vi "Save param in PGserver.vi"(4 "Param row name 2":string, 6 "Param row name1":string, 7 "conninfo":T1={"host"="localhost", "port"="5432", "client_encoding"="WIN1251", "dbname"="system", "user"="postgres", "password"=""}, 8 "error in (no error)":errorcluster, 9 "Param column Name":string="value", 10 "Param Table":string="par", 11 "Parameter":string) -> (0 "error out":errorcluster)   [LabVIEW 2019, in "PostgreSQL.lvlib"]
uses:
  PostgreSQL.lvlib
  ctl/Coninfo.ctl
  PostgreSQL2LabVIEW/libpqlv/src/PQresultErrorMessage.vi
  PostgreSQL2LabVIEW/libpqUtility/src/PQclear.vi
  PostgreSQL2LabVIEW/libpqlv/src/PQsendQuery.vi
  PostgreSQL2LabVIEW/libpqlv/src/PQgetResult.vi
  PostgreSQL2LabVIEW/libpqlv/src/PQresultStatus.vi
  PostgreSQL2LabVIEW/libpqlv/src/PQfinish.vi
  PostgreSQL2LabVIEW/libpqlv/src/PQconnectdb.vi
  PostgreSQL2LabVIEW/libpqlv/src/PQerrorMessage.vi
  PostgreSQL2LabVIEW/libpqlv/src/PQstatus.vi
  <vilib>/dlg_ctls.llb/Space Constant.vi
  PostgreSQL2LabVIEW/libpqlv/src/PQclear.vi
  PostgreSQL2LabVIEW/libpqUtility/libpqutility.lvlib
  PostgreSQL2LabVIEW/libpqUtility64/libpqutility64.lvlib
panel:
  out "PQStatus":T2(ring)
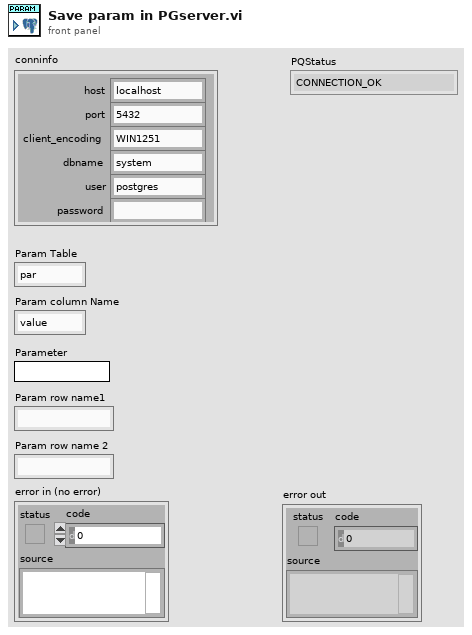
[diagram p1: front panel]
types:
  T1 = typedef "PostgreSQL.lvlib/Coninfo.ctl" = cluster{"host":string, "port":string, "client_encoding":string, "dbname":string, "user":string, "password":string}
  T2 = enum32{"CONNECTION_OK", "CONNECTION_BAD", "CONNECTION_STARTED", "CONNECTION_MADE", "CONNECTION_AWAITING_RESPONSE", "CONNECTION_AUTH_OK", "CONNECTION_SETENV", "CONNECTION_SSL_STARTUP", "CONNECTION_NEEDED"}
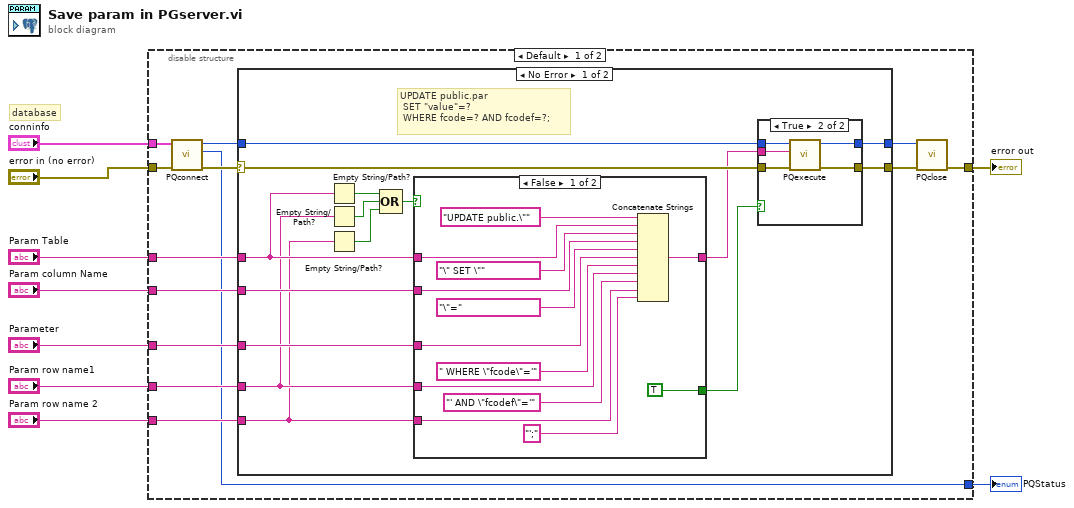
[diagram p0: block diagram]
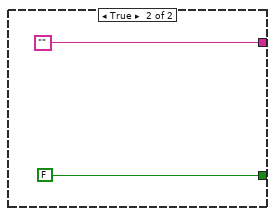
[diagram p2: hidden frame]
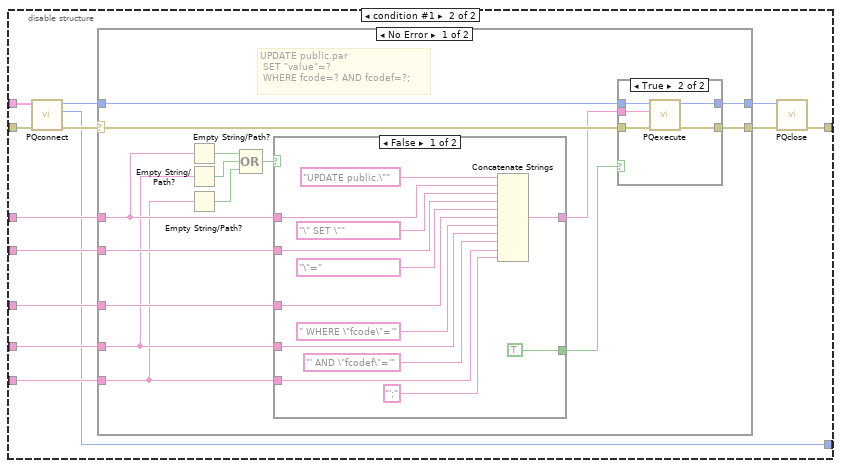
[diagram p5: hidden frame]
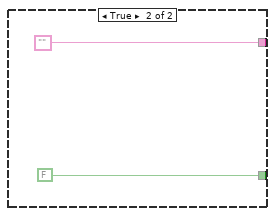
[diagram p6: hidden frame]
diagram:
  # "database"
  n1 = disable-structure shown="Default" {
    disable-tunnel: "Parameter" -> [w20 w66]
    disable-tunnel: [w18 w62] -> w8
    disable-tunnel: "conninfo" -> [w17 w70]
    disable-tunnel: "Param row name1" -> [w15 w65]
    disable-tunnel: "Param Table" -> [w14 w68]
    disable-tunnel: "Param column Name" -> [w13 w67]
    disable-tunnel: "Param row name 2" -> [w12 w64]
    disable-tunnel: "error in (no error)" -> [w11 w69]
    disable-tunnel: [w10 w63] -> w1
    frame condition #0 (active) {
      n2 = call "PQconnect.vi"("error in (no error)"=w11, "conninfo"=w17) -> ("error out"=w22:errorcluster, "PQStatus"=w10:T2, "conn"=w21:u32)  [unwired: 7 in]
      n3 = case shown="No Error" w22 {
        selector: w22 -> [w37 w61]
        tunnel: w20 -> [w36 _]
        tunnel: w21 -> [w35 w60]
        tunnel: w14 -> [w34 _]
        tunnel: [w33 w61] -> w16
        tunnel: w15 -> [w26 _]
        tunnel: w13 -> [w28 _]
        tunnel: w12 -> [w25 _]
        tunnel: [w23 w60] -> w19
        frame No Error {
          # "UPDATE public.par\n\tSET \"value\"=?\n\tWHERE fcode=? AND fcodef=?;"
          n4 = Empty String/Path?(string/path=w34) -> (empty?=w32:bool)
          n5 = Empty String/Path?(string/path=w26) -> (empty?=w27:bool)
          n6 = Empty String/Path?(string/path=w25) -> (empty?=w24:bool)
          n7 = Compound Arithmetic op=OR(w32, w27, w24) -> (w31:bool)
          n8 = case shown="False" w31 {
            tunnel: [w49 ""] -> w30
            tunnel: w34 -> [w47 _]
            tunnel: [TRUE FALSE] -> w29
            tunnel: w26 -> [w40 _]
            tunnel: w36 -> [w38 _]
            tunnel: w28 -> [w42 _]
            tunnel: w25 -> [w39 _]
            frame False {
              n9 = Concatenate Strings("UPDATE public.\"" ("table"), w47, "\" SET \"" ("table"), w42, "\"=" ("table"), w38, " WHERE \"fcode\"='" ("string"), w40, "' AND \"fcodef\"='" ("string"), w39, "';" ("string")) -> (w49:string)
            }
            frame True {
            }
          }
          n10 = case shown="True" w29 {
            tunnel: w37 -> [w54 w59]
            tunnel: w35 -> [w53 w57]
            tunnel: w30 -> [_ w58]
            tunnel: [w54 w56] -> w33
            tunnel: [w53 w55] -> w23
            frame False {
            }
            frame True {
              n11 = call "PQexecute.vi"("error in"=w59, "SQL querry"=w58, "conn"=w57) -> ("error out"=w56:errorcluster, "conn_out"=w55:u32)  [unwired: 7 in]
            }
          }
        }
        frame Error {
        }
      }
      n12 = call "PQclose.vi"("error in (no error)"=w16, "conn"=w19) -> ("error out"=w18:errorcluster)  [unwired: 9 in]
    }
    frame condition #1 {
      n13 = call "PQconnect.vi"("error in (no error)"=w69, "conninfo"=w70) -> ("error out"=w74:errorcluster, "PQStatus"=w63:T2, "conn"=w73:u64)  [unwired: 7 in]
      n14 = case shown="No Error" w74 {
        selector: w74 -> [w89 w113]
        tunnel: w66 -> [w88 _]
        tunnel: w73 -> [w87 w112]
        tunnel: w68 -> [w86 _]
        tunnel: [w85 w113] -> w71
        tunnel: w65 -> [w78 _]
        tunnel: w67 -> [w80 _]
        tunnel: w64 -> [w77 _]
        tunnel: [w75 w112] -> w72
        frame No Error {
          # "UPDATE public.par\n\tSET \"value\"=?\n\tWHERE fcode=? AND fcodef=?;"
          n15 = Empty String/Path?(string/path=w86) -> (empty?=w84:bool)
          n16 = Empty String/Path?(string/path=w78) -> (empty?=w79:bool)
          n17 = Empty String/Path?(string/path=w77) -> (empty?=w76:bool)
          n18 = Compound Arithmetic op=OR(w84, w79, w76) -> (w83:bool)
          n19 = case shown="False" w83 {
            tunnel: [w101 ""] -> w82
            tunnel: w86 -> [w99 _]
            tunnel: [TRUE FALSE] -> w81
            tunnel: w78 -> [w92 _]
            tunnel: w88 -> [w90 _]
            tunnel: w80 -> [w94 _]
            tunnel: w77 -> [w91 _]
            frame False {
              n20 = Concatenate Strings("UPDATE public.\"" ("table"), w99, "\" SET \"" ("table"), w94, "\"=" ("table"), w90, " WHERE \"fcode\"='" ("string"), w92, "' AND \"fcodef\"='" ("string"), w91, "';" ("string")) -> (w101:string)
            }
            frame True {
            }
          }
          n21 = case shown="True" w81 {
            tunnel: w89 -> [w106 w111]
            tunnel: w87 -> [w105 w109]
            tunnel: w82 -> [_ w110]
            tunnel: [w106 w108] -> w85
            tunnel: [w105 w107] -> w75
            frame False {
            }
            frame True {
              n22 = call "PQexecute.vi"("error in"=w111, "SQL querry"=w110, "conn"=w109) -> ("error out"=w108:errorcluster, "conn_out"=w107:u64)  [unwired: 7 in]
            }
          }
        }
        frame Error {
        }
      }
      n23 = call "PQclose.vi"("error in (no error)"=w71, "conn"=w72) -> ("error out"=w62:errorcluster)  [unwired: 9 in]
    }
  }
  "error out" <- w8
  "PQStatus" <- w1
